vi "ESP301.vi"() -> ()   [LabVIEW 2019]
uses:
  Desktop/Manip_uPL_visible_2020/SubVIs/ExistingSetupVIs/GH014/Labview/ESP 301/Newport ESP301/Newport ESP301.lvlib
panel:
  in  "Turn Motor On":bool
  in  "stop":bool
  in  "milliseconds to wait":u32
  in  "Numeric":i32
  out "Units":T1(ring)
  out "AXIS":i32
  out "Motor Type (Undefined)":T2(ring)
  in  "Serial Link (RS232)":enum16{"RS232", "USB"}(ring)=enum."USB"
  out "Motor Status":bool
  in  "ESP 301 COM Port":refnum<visa-resource-name>="ASRL4::INSTR"
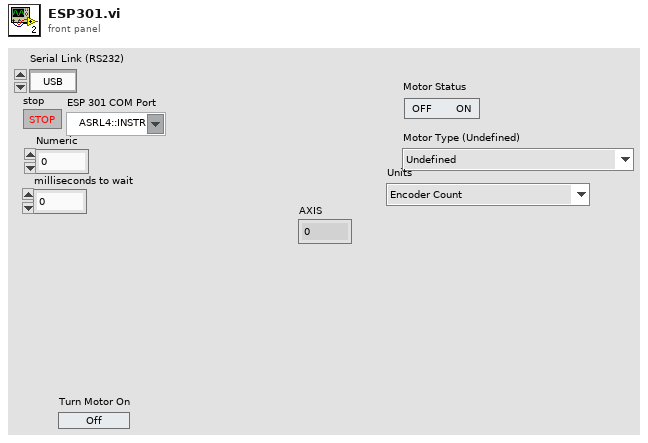
[diagram p1: front panel]
types:
  T1 = enum16{"Encoder Count", "Motor Step", "millimeter", "micrometer", "inch", "milli-inch", "micro-inch", "degree", "gradian", "radian", "milliradian", "microradian"}
  T2 = enum16{"Undefined", "DC Servo Motor", "Step Motor (not supported)", "Commutated Step Motor", "Commutate Brushless DC Servo Motor"}
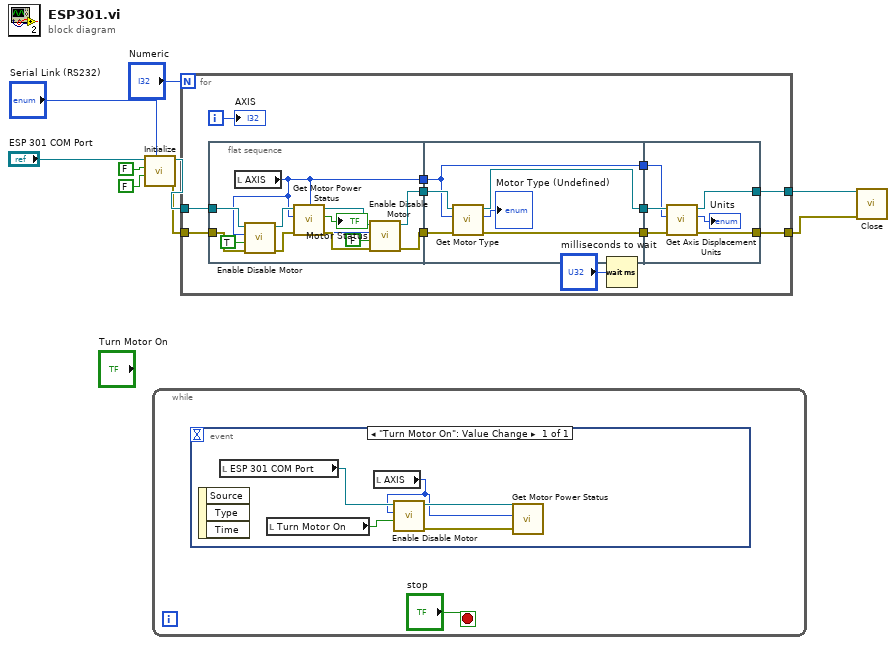
[diagram p0: block diagram]
diagram:
  n1 = call "Initialize.vi"("VISA resource name"="ESP 301 COM Port", "ID Query (True)"=FALSE, "Reset (False)"=FALSE, "Serial Link (RS232)"="Serial Link (RS232)") -> ("VISA resource name out"=w8:refnum<visa-resource-name>, "error out"=w7:errorcluster)  [unwired: 5 in]
  n2 = while {
    stop <- "stop" stop-if-true
    n3 = event shown="[0] \"Turn Motor On\": Value Change" {
      selector: _ -> [_]
      dyn-events: _ -> [_]
      timeout: _ -> [_]
      event "Turn Motor On": Value Change {
        n4 = event-data() -> ()  [unwired: 1 in, 3 out]
        n5 = local read "ESP 301 COM Port"() -> (w15:refnum<visa-resource-name>)
        n6 = local read "Turn Motor On"() -> (w14:bool)
        n7 = local read "AXIS"() -> (w11:i32)
        n8 = call "Enable Disable Motor.vi"("Action (F - OFF)"=w14, "Axis (1)"=w11, "VISA resource name"=w15) -> ("error out"=w12:errorcluster, "VISA resource name out"=w13:refnum<visa-resource-name>)  [unwired: 3 in]
        n9 = call "Get Motor Power Status.vi"("error in (no error)"=w12, "Axis (1)"=w11, "VISA resource name"=w13) -> ()  [unwired: 2 in, 3 out]
      }
    }
  }
  n10 = for {
    N: "Numeric" -> [_]
    tunnel: w8 -> [w22]
    tunnel: w7 -> [w21]
    tunnel: [w20] -> w3
    tunnel: [w17] -> w2
    i -> [w19]
    n11 = flat-sequence {
      tunnel: w22 -> [w37]
      tunnel: w21 -> [w38]
      tunnel: [w33] -> w27
      tunnel: [w32] -> w26
      tunnel: [w29] -> w25
      tunnel: w27 -> [w45]
      tunnel: w26 -> [w44]
      tunnel: w25 -> [w40]
      tunnel: [w42] -> w24
      tunnel: [w43] -> w23
      tunnel: [w40] -> w18
      tunnel: [w46] -> w20
      tunnel: w24 -> [w50]
      tunnel: w23 -> [w51]
      tunnel: w18 -> [w49]
      tunnel: [w47] -> w17
      frame #0 {
        n12 = local read "AXIS"() -> (w29:i32)
        n13 = call "Enable Disable Motor.vi"("error in (no error)"=w38, "Action (F - OFF)"=TRUE, "Axis (1)"=w29, "VISA resource name"=w37) -> ("error out"=w35:errorcluster, "VISA resource name out"=w36:refnum<visa-resource-name>)  [unwired: 2 in]
        n14 = call "Get Motor Power Status.vi"("error in (no error)"=w35, "Axis (1)"=w29, "VISA resource name"=w36) -> ("error out"=w30:errorcluster, "Power Status"=→"Motor Status":bool, "VISA resource name out"=w31:refnum<visa-resource-name>)  [unwired: 2 in]
        n15 = call "Enable Disable Motor.vi"("error in (no error)"=w30, "Action (F - OFF)"=FALSE, "Axis (1)"=w29, "VISA resource name"=w31) -> ("error out"=w33:errorcluster, "VISA resource name out"=w32:refnum<visa-resource-name>)  [unwired: 2 in]
      }
      frame #1 {
        n16 = call "Get Motor Type.vi"("error in (no error)"=w45, "Axis (1)"=w40, "VISA resource name"=w44) -> ("error out"=w42:errorcluster, "Motor Type (Undefined)"=→"Motor Type (Undefined)":T2, "VISA resource name out"=w43:refnum<visa-resource-name>)  [unwired: 2 in]
      }
      frame #2 {
        n17 = call "Get Axis Displacement Units.vi"("error in (no error)"=w50, "Axis (1)"=w49, "VISA resource name"=w51) -> ("error out"=w47:errorcluster, "Units"=→"Units":T1, "VISA resource name out"=w46:refnum<visa-resource-name>)  [unwired: 2 in]
      }
    }
    n18 = Wait (ms)(milliseconds to wait="milliseconds to wait") -> ()  [unwired: 1 out]
    "AXIS" <- w19
  }
  n19 = call "Close.vi"("error in (no error)"=w2, "VISA resource name"=w3) -> ()  [unwired: 9 in, 1 out]
